vi "AlliGator Get-Set Skippable Dialog.vi"(6 "Set/Get (F)":bool, 8 "Error In":errorcluster, 9 "Is skipped (in)":bool, 11 "Dialog Window VI Name":string) -> (0 "Error Out":errorcluster, 1 "Is skipped (out)":bool)   [LabVIEW 2021, in "AlliGator GUI.lvlib"]
doc: "Stores state of dialog windows with a \"Skip this dialog in the future\" checkbox."
uses:
  AlliGator GUI.lvlib
  Globals, Variables, Constants/AlliGator Variables List.ctl
  AlliGator Skippable Windows Status.ctl
  Globals, Variables, Constants/AlliGator Globals, Variables & Constants.lvlib
panel:
  # "see the AlliGator License on the block diagram (Ctrl+E or Window:Show Block Diagram)"
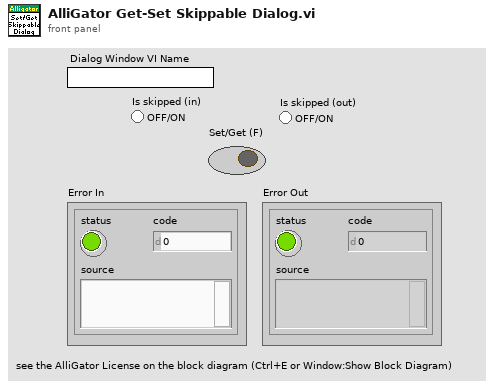
[diagram p1: front panel]
types:
  T1 = typedef "AlliGator GUI.lvlib/AlliGator Skippable Windows Status.ctl" = cluster{"Dialog Window Name":string, "Is skipped":bool}
  T2 = typedef "AlliGator Globals, Variables & Constants.lvlib/AlliGator Variables List.ctl" = enum16{"---- GUI ----", "GUI:Initialization Status", "GUI:State Indicators Refnum", "GUI:Original AlliGator Menu Items", "GUI:Current Action Loop State", "GUI:Script in progress", "GUI:Playback", "GUI:Loop Playback", "GUI:Search ROI Used", "GUI:Search ROI", "Decay Graph Max Legend Size", "Intensity Graph Max Legend Size", "Decay Statistics Graph Max Legend Size", "Phasor Graph Max Legend Size", "Phasor Ratio Graph Max Legend Size", "Lifetime Graph Max Legend Size", "---- Files ----", "Files:Export Dataset Frames as Individual Files", "Files:Show Batch Export Help Balloons", "Files:Frames in Dataset", "Files:ptu File Frame Start Indices", "Files:Current Frame in Dataset", "Files:Current Frame Timestamp", "Files:Dataset Loaded", "Files:Dataset Metadata", "Files:Dataset Channel", "Files:Dataset Data Description", "Files:Background Dataset Metadata", "Files:Background Dataset Channel", "Files:Background Dataset Data Description", "Files:Background File Subtraction", "Files:Background File Path", "Files:Background File Pile-up Correction", "Files:Background File Pixel Well Capacity", "Files:Background File Scaling Factor", "Files:Current Dataset Load Settings", "Files:Dataset Path", "Files:ICCD-specific Information", "Files:Macrotime Gate Separation", "------ Python Plugins ------", "Python Plugins:Information", "Python Plugins:Python Session", "Python Plugins:Valid Python Session?", "---- Source Image ----", "Source Image:ROIs", "Source Image:Current ROI", "Source Image:ROI Event Refnum", "X_Source Image Display Range", "X_Source Image Palette Information", "X_Type of Displayed Image", "X_Time Gate Slider", "Source Image:Palette List", "Source Image:Scale", "Source Image:ROI Overlay Color", "Source Image:Overlay to Erase", "Source Image:Is Displayed Image Accumulated", "Source Image:White Light Image Modified", "Source Image:Mask Image Modified", "---- Image Profile Window ----", "Image Profile:Window Event Refnum", "Image Profile:IntensityType", "Image Profile:Intensity Average Type", "Image Profile:Intensity-weighted SDV", "Image Profile:Box Profile Type", "Image Profile:Window Open", "Image Profile:Plotted Fit Parameter", "------ Phasor Graph -------", "Phasor Graph:Show Line", "---- Phasor Plot ---", "Phasor Plot:Parameters Changed", "Phasor Plot:FLI Dataset Modified since last Calculation", "Phasor Harmonics Data", "Selected Phasor Harmonics", "Phasor Harmonic Manager Event Refnum", "Phasor Plot:ROIs", "Phasor Plot:Current ROI", "Phasor Plot:ROI Event Refnum", "Phasor Plot:Image Reference Points", "Phasor Plot:Computed", "Phasor Plot:Palette Information", "Phasor Plot:Palette List", "Phasor Plot:Phasor Ratio Palette Information", "Phasor Plot:Phasor Ratio Palette List", "Phasor Plot:Image Scale", "Phasor Plot:Image Overlay to Erase", "Phasor Plot:Image Elements to Update", "Phasor Plot:Current Calculation Parameters", "Phasor Plot:Current Calibration Options", "Phasor Plot:Reset Cumulated Phasor Plot", "Phasor Plot:Reference 1", "Phasor Plot:Lifetime Reference 1", "Phasor Plot:Reference 1 Frequency", "Phasor Plot:Reference 2", "Phasor Plot:Lifetime Reference 2", "Phasor Plot:Reference 2 Frequency", "---- Decay Analysis ----", "Number of Selected Decays to Fit", "LS Fit Results", "LAR Fit Results", "BS Fit Results", "Last Decay Max - Min", "Best Fit Parameters", "Best Fit Parameter Names", "Actual Size X", "Actual Size Y", "Binning X", "Binning Y", "Actual # Gates", "Dataset Number", "Gates to...", "Gates Skipped", "Gates to keep", "Gate Step", "Gate Separation", "Reversed Gates", "Pile-up Correction", "Pixel Well Capacity", "Background Subtracted", "Background Subtraction Method", "Background Definition Range", "Background File (deprecated)", "Number of Dataset Accumulated", "Array of Accumulated Dataset Paths", "Do Averaged Datasets", "Destination File Path", "Process Plot Target", "Use 1/D as Phasor Frequency", "---- Decay Fit Parameter Map -----", "Decay Fit Parameter Map:Palette Information", "Decay Fit Parameter Map:Palette List", "---- Parameter Map ----", "Parameter Map:Palette Information", "Parameter Map:Palette List", "------- Local Decay Window ---------", "Local Decay Graph Window:Event Refnum", "Local Decay Graph Window:Use normalized IRF for convolution", "----- Miscellaneous ----", "Misc:Skippable Dialog Windows Status"}
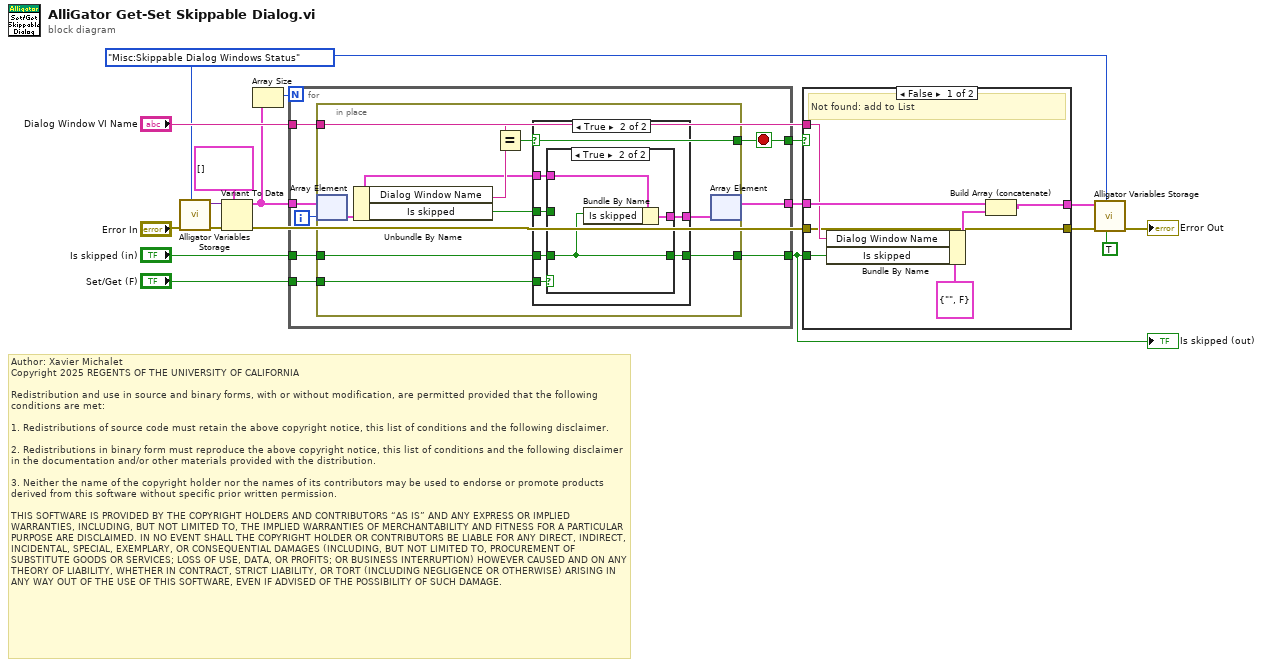
[diagram p0: block diagram]
diagram:
  w1 = AlliGator_Variables_List."Misc:Skippable Dialog Windows Status" ("Alligator Variable")
  # "Author: Xavier Michalet\nCopyright 2025 REGENTS OF THE UNIVERSITY OF CALIFORNIA\n\nRedistribution and use in source and binary forms, with or without modification, are permitted provided that the following conditions are met:\n\n1. Redistributions of source code must retain the above copyright notice, this list of conditions and the following disclaimer.\n\n2. Redistributions in binary form must reproduce the above copyright notice, this list of conditions and the following disclaimer in the documentation and/or other materials provided with the distribution.\n\n3. Neither the name of the copyright holder nor the names of its contributors may be used to endorse or promote products derived from this software without specific prior written permission.\n\nTHIS SOFTWARE IS PROVIDED BY THE COPYRIGHT HOLDERS AND CONTRIBUTORS “AS IS” AND ANY EXPRESS OR IMPLIED WARRANTIES, INCLUDING, BUT NOT LIMITED TO, THE IMPLIED WARRANTIES OF MERCHANTABILITY AND FITNESS FOR A PARTICULAR PURPOSE ARE DISCLAIMED. IN NO EVENT SHALL THE COPYRIGHT HOLDER OR CONTRIBUTORS BE LIABLE FOR ANY DIRECT, INDIRECT, INCIDENTAL, SPECIAL, EXEMPLARY, OR CONSEQUENTIAL DAMAGES (INCLUDING, BUT NOT LIMITED TO, PROCUREMENT OF SUBSTITUTE GOODS OR SERVICES; LOSS OF USE, DATA, OR PROFITS; OR BUSINESS INTERRUPTION) HOWEVER CAUSED AND ON ANY THEORY OF LIABILITY, WHETHER IN CONTRACT, STRICT LIABILITY, OR TORT (INCLUDING NEGLIGENCE OR OTHERWISE) ARISING IN ANY WAY OUT OF THE USE OF THIS SOFTWARE, EVEN IF ADVISED OF THE POSSIBILITY OF SUCH DAMAGE."
  n1 = call "Alligator Variables Storage.vi"("AlliGator Variable"=w1, "Error In"="Error In") -> ("Error Out"=w17:errorcluster, "Data out"=w16:variant)  [unwired: 7 in, 1 out]
  n2 = Variant To Data(error in=w17, type=T1[] [], Variant=w16) -> (data=w8:T1[], error out=w6:errorcluster)
  n3 = Array Size(array=w8) -> (size(s)=w7:i32)
  n4 = for {
    N: w7 -> [_]
    tunnel: w8 -> [w23]
    tunnel: "Dialog Window VI Name" -> [w26]
    tunnel: [w24] -> w9
    tunnel: "Set/Get (F)" -> [w25]
    tunnel: "Is skipped (in)" -> [w21]
    tunnel: [w20] -> w11
    tunnel: [w19] -> w12
    i -> [w22]
    stop <- w19 stop-if-true
    n5 = in-place {
      in-place-border: w26 -> [w34]
      in-place-border: [w27] -> w19
      in-place-border: w25 -> [w33]
      in-place-border: [w31] -> w24
      in-place-border: w21 -> [w28]
      n6 = in-place-array #1(w23, w22) -> (w30:T1)
      n7 = Unbundle By Name(w30) -> ("Dialog Window Name"=w35:string, "Is skipped"=w32:bool)
      n8 = Equal?(x=w34, y=w35) -> (x = y?=w27:bool)
      n9 = case shown="True" w27 {
        tunnel: w33 -> [_ w43]
        tunnel: w32 -> [_ w42]
        tunnel: [w36 w41] -> w31
        tunnel: w30 -> [w37 w40]
        tunnel: [w37 w39] -> w29
        tunnel: w28 -> [w36 w38]
        frame False {
        }
        frame True {
          n10 = case shown="True" w43 {
            tunnel: w42 -> [w45 _]
            tunnel: [w45 w46] -> w41
            tunnel: w40 -> [w44 w48]
            tunnel: [w44 w47] -> w39
            tunnel: w38 -> [_ w46]
            frame False {
            }
            frame True {
              n11 = Bundle By Name(cluster=w48, "Is skipped"=w46) -> (w47:T1)
            }
          }
        }
      }
      n12 = in-place-array #1(w29) -> (w20:T1[])  [unwired: 1 out]
    }
  }
  "Is skipped (out)" <- w9
  n13 = case shown="False" w12 {
    tunnel: w11 -> [w55 w56]
    tunnel: "Dialog Window VI Name" -> [w54 _]
    tunnel: w9 -> [w53 _]
    tunnel: [w49 w57] -> w4
    tunnel: w6 -> [w49 w57]
    tunnel: [w50 w56] -> w5
    frame False {
      # "Not found: add to List"
      n14 = Bundle By Name(cluster=T1 {"Dialog Window Name"="", "Is skipped"=FALSE} ("Skippable Dialog Windows Status"), "Dialog Window Name"=w54, "Is skipped"=w53) -> (w51:T1)
      n15 = Build Array (concatenate)(w55, w51) -> (w50:T1[])
    }
    frame True {
      # "Found"
    }
  }
  n16 = call "Alligator Variables Storage.vi"("Get(F)/Set"=TRUE, "AlliGator Variable"=w1, "Error In"=w4, "Data in"=w5) -> ("Error Out"=→"Error Out":errorcluster)  [unwired: 5 in, 2 out]
